vi "Configure Serial Bus (I2S - Source).vi"(0 "VISA resource name":refnum<visa-resource-name>, 1 "Data Source Channel (0: Channel 1)":i32(ring) items=["Channel 1"=0, "Channel 2"=1, "Channel 3"=2, "Channel 4"=3, "D0"=13, "D1"=14, "D2"=15, "D3"=16, "D4"=17, "D5"=18, "D6"=19, "D7"=20, "D8"=21, "D9"=22, "D10"=23, "D11"=24, "D12"=25, "D13"=26, "D14"=27, "D15"=28, "External"=29], 5 "Serial Bus Name (1: Serial Bus 1)":i32(ring)=1 items=["Serial Bus 1"=1, "Serial Bus 2"=2], 9 "WS Source Channel (1: Channel 2)":i32(ring)=1 items=["Channel 1"=0, "Channel 2"=1, "Channel 3"=2, "Channel 4"=3, "D0"=13, "D1"=14, "D2"=15, "D3"=16, "D4"=17, "D5"=18, "D6"=19, "D7"=20, "D8"=21, "D9"=22, "D10"=23, "D11"=24, "D12"=25, "D13"=26, "D14"=27, "D15"=28, "External"=29], 11 "error in (no error)":errorcluster, 12 "Clock Source Channel (1: Channel 2)":i32(ring)=1 items=["Channel 1"=0, "Channel 2"=1, "Channel 3"=2, "Channel 4"=3, "D0"=13, "D1"=14, "D2"=15, "D3"=16, "D4"=17, "D5"=18, "D6"=19, "D7"=20, "D8"=21, "D9"=22, "D10"=23, "D11"=24, "D12"=25, "D13"=26, "D14"=27, "D15"=28, "External"=29]) -> (4 "VISA resource name out":refnum<visa-resource-name>, 15 "error out":errorcluster)   [LabVIEW 2016, in "Agilent 2000 3000 X-Series.lvlib"]
doc: "Configures the source settings of I2S bus."
uses:
  Agilent 2000 3000 X-Series.lvlib
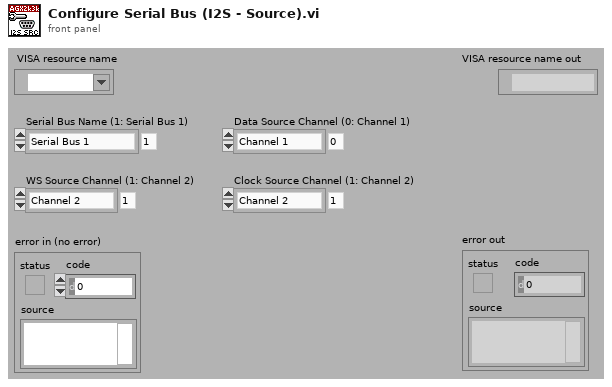
[diagram p1: front panel]
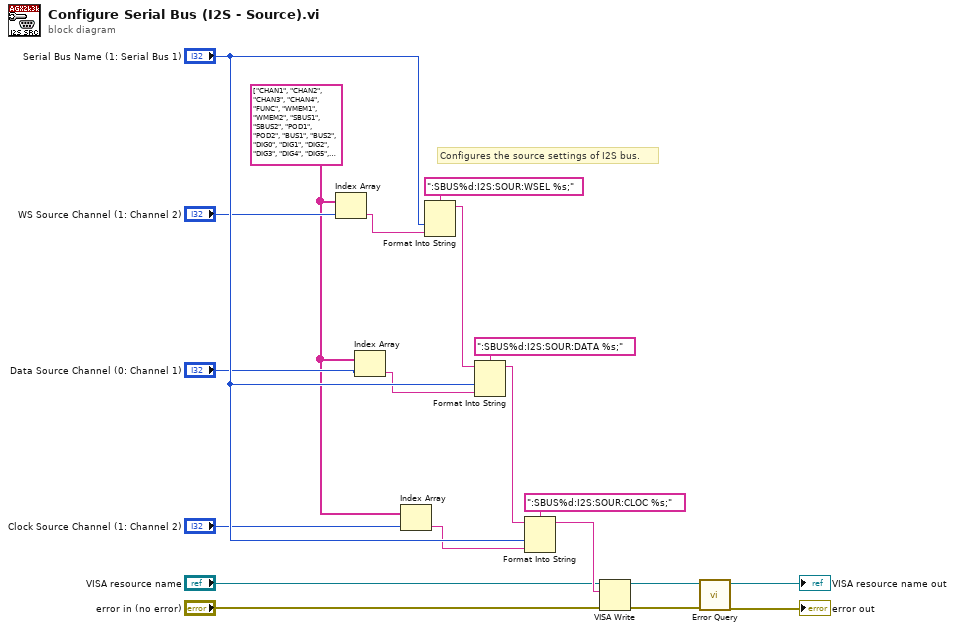
[diagram p0: block diagram]
diagram:
  w3 = string[] ["CHAN1", "CHAN2", "CHAN3", "CHAN4", "FUNC", "WMEM1", "WMEM2", "SBUS1", "SBUS2", "POD1", "POD2", "BUS1", "BUS2", "DIG0", "DIG1", "DIG2", "DIG3", "DIG4", "DIG5", "DIG6", "DIG7", "DIG8", "DIG9", "DIG10", "DIG11", "DIG12", "DIG13", "DIG14", "DIG15", "EXT", "LINE", "WGEN"]
  # "Configures the source settings of I2S bus."
  n1 = Index Array(array=w3, index="WS Source Channel (1: Channel 2)") -> (element=w6:string)
  n2 = Index Array(array=w3, index="Data Source Channel (0: Channel 1)") -> (element=w5:string)
  n3 = Index Array(array=w3, index="Clock Source Channel (1: Channel 2)") -> (element=w2:string)
  n4 = Format Into String(format string=":SBUS%d:I2S:SOUR:WSEL %s;", "Serial Bus Name (1: Serial Bus 1)", w6) -> (resulting string=w18:string)  [unwired: 2 in, 1 out]
  n5 = Format Into String(format string=":SBUS%d:I2S:SOUR:DATA %s;", initial string=w18, "Serial Bus Name (1: Serial Bus 1)", w5) -> (resulting string=w16:string)  [unwired: 1 in, 1 out]
  n6 = Format Into String(format string=":SBUS%d:I2S:SOUR:CLOC %s;", initial string=w16, "Serial Bus Name (1: Serial Bus 1)", w2) -> (resulting string=w14:string)  [unwired: 1 in, 1 out]
  n7 = VISA Write(VISA resource name="VISA resource name", write buffer=w14, error in (no error)="error in (no error)") -> (VISA resource name out=w11:refnum<visa-resource-name>, error out=w10:errorcluster)  [unwired: 1 out]
  n8 = call "Error Query.vi"("error in (no error)"=w10, "VISA resource name"=w11) -> ("error out"=→"error out":errorcluster, "VISA resource name out"=→"VISA resource name out":refnum<visa-resource-name>)  [unwired: 8 out]
